vi "SwissSPAD Live_Pre-Recording Checks.vi"(8 "error in (no error)":errorcluster, 9 "Init Series?":bool, 11 "SwissSPAD Live Internal Variables in":T1={"okCFrontPanelDevices Refnum"=refnum, "Bottom Device Refnum"=refnum, "Display Image"=refnum, "# Live Images"=0, "relative s"=0.0, "# Image Sets"=0, "Message"="", "Current Image Set"=0, "# Datasets in Series"=0, "Current Dataset"=0, "Live Mode"=FALSE, "Recording Mode"=FALSE, "Record Button"=refnum, "\nLive Button"=refnum, "SwissSPAD Live Gate Image Data Q Name"="SS2 Live Gate Data Q", "Discard First Image"=FALSE, "Image Information"={"Save ROI Only"=FALSE, "Left"=0, "Top"=0, "Right"=0, "Bottom"=0, "Use Current ROI"=FALSE}, "Image Binning Options"={"Use Image Binning"=FALSE, "X Bin"=1, "Y Bin"=1}, "Bottom FPGA Serial Number"="", "Detector PCB Version"=enum."SS2 PCB1", "# Acquisitions"=1, "10 bits"=FALSE, "Top FPGA Serial Number"="", "Top Device Refnum"=refnum, "okCFrontPanel Refnum"=refnum} {"# Acquisitions" min=1; "Image Binning Options"."Y Bin" min=1; "Image Binning Options"."X Bin" min=1}) -> (0 "error out":errorcluster, 1 "Message":string, 2 "Ready?":bool, 3 "SwissSPAD Live Internal Variables out":T1={"okCFrontPanelDevices Refnum"=refnum, "Bottom Device Refnum"=refnum, "Display Image"=refnum, "# Live Images"=0, "relative s"=0.0, "# Image Sets"=0, "Message"="", "Current Image Set"=0, "# Datasets in Series"=0, "Current Dataset"=0, "Live Mode"=FALSE, "Recording Mode"=FALSE, "Record Button"=refnum, "\nLive Button"=refnum, "SwissSPAD Live Gate Image Data Q Name"="SS2 Live Gate Data Q", "Discard First Image"=FALSE, "Image Information"={"Save ROI Only"=FALSE, "Left"=0, "Top"=0, "Right"=0, "Bottom"=0, "Use Current ROI"=FALSE}, "Image Binning Options"={"Use Image Binning"=FALSE, "X Bin"=1, "Y Bin"=1}, "Bottom FPGA Serial Number"="", "Detector PCB Version"=enum."SS2 PCB1", "# Acquisitions"=1, "10 bits"=FALSE, "Top FPGA Serial Number"="", "Top Device Refnum"=refnum, "okCFrontPanel Refnum"=refnum} {"# Acquisitions" min=1; "Image Binning Options"."Y Bin" min=1; "Image Binning Options"."X Bin" min=1}, 4 "Verbose Message":string)   [LabVIEW 2021]
uses:
  SwissSPAD Live_Internal Variables.ctl
  D:/UCLA Thinkpad Google Drive/LabVIEW 2021 SP1/builds/SwissSPAD Live Distribution/Opal Kelly/C# Wrapper/v5.0.2/libFrontPanel-csharp.dll
  Opal Kelly/C# Wrapper/v5.0.2/libFrontPanel-csharp.dll
  <vilib>/vision/Image Controls.llb/IMAQ Image.ctl
  SwissSPAD Live_Image ROI Information.ctl
  Phasor/Image Binning Options.ctl
  SwissSPAD Live_SSx PCB Version.ctl
  SwissSPAD Live_Settings List.ctl
  SwissSPAD Live_File Information.ctl
  SwissSPAD Live_Globals.vi
  Variant/Variant to Data/Variant to Data.lvlib
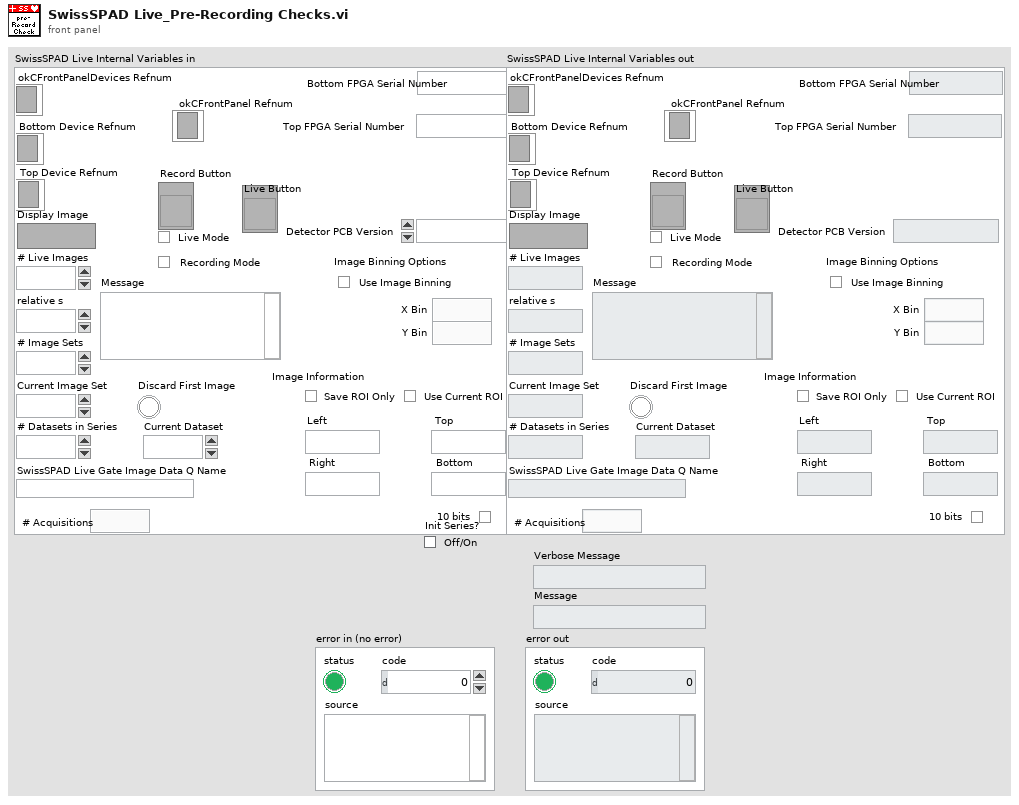
[diagram p1: front panel]
types:
  T1 = typedef "SwissSPAD Live_Internal Variables.ctl" = cluster{"okCFrontPanelDevices Refnum":refnum<k24>, "Bottom Device Refnum":refnum<k24>, "Display Image":T2, "# Live Images":i32, "relative s":dbl, "# Image Sets":i32, "Message":string, "Current Image Set":i32, "# Datasets in Series":i32, "Current Dataset":i32, "Live Mode":bool, "Recording Mode":bool, "Record Button":refnum<vi>, "\nLive Button":refnum<vi>, "SwissSPAD Live Gate Image Data Q Name":string, "Discard First Image":bool, "Image Information":T3, "Image Binning Options":T4, "Bottom FPGA Serial Number":string, "Detector PCB Version":T5, "# Acquisitions":u32, "10 bits":bool, "Top FPGA Serial Number":string, "Top Device Refnum":refnum<k24>, "okCFrontPanel Refnum":refnum<k24>}
  T2 = typedef "IMAQ Image.ctl" = refnum<image>
  T3 = typedef "SwissSPAD Live_Image ROI Information.ctl" = cluster{"Save ROI Only":bool, "Left":u16, "Top":u16, "Right":u16, "Bottom":u16, "Use Current ROI":bool}
  T4 = typedef "Image Binning Options.ctl" = cluster{"Use Image Binning":bool, "X Bin":i32, "Y Bin":i32}
  T5 = typedef "SwissSPAD Live_SSx PCB Version.ctl" = enum16{"unknown", "SS2 PCB1", "SS2 PCB2", "SS3 PCB1"}
  T6 = typedef "SwissSPAD Live_Settings List.ctl" = enum16{"FPGA:Bottom Half", "FPGA:Top Half", "FPGA:Bottom Bitfile Path", "FPGA:Top Bitfile Path", "FPGA:Bottom Bitstream Version", "FPGA:Top Bitstream Version", "FPGA:Auto Reset FPGA", "FPGA:Bottom FPGA Serial Number", "FPGA:Top FPGA Serial Number", "FPGA:Detector PCB Version", "Acquisition Parameters:Microlens", "Acquisition Parameters:SS2 DAQ Parameters", "Acquisition Parameters:Gate Configuration Array", "Acquisition Parameters:SS3 DAQ Parameters", "Acquisition Parameters:Buffer Size (# 8-bit Gates)", "File Information:File Information", "File Information:# Datasets in Series", "File Information:Scrambled File Flag", "File Information:SS3 Gate Slip Correction", "File Information:SS3 Hot Pixel Mismatch Detection", "File Information:Delay between Datasets", "File Information:Save Sum of All Gates Preview", "Image Parameters:Image ROI Information", "Image Parameters:Image Binning Options", "Image Parameters:SS3 Displayed Image", "Image Parameters:Image Display Options", "Image Parameters:Use Histogram Cursors", "Image Parameter:FPGA Data to Display", "UI Settings:Histogram Bins Number", "UI Settings:Histogram Bin Size", "UI Settings:Use Image Display Options", "UI Settings:Verbose Settings", "UI Settings:Verbose Saving"}
  T7 = typedef "SwissSPAD Live_File Information.ctl" = cluster{"File Folder":path, "File Name":string, "File Index":u32, "Author":string, "Sample":string, "Compression":bool, "Compression Level":u8}
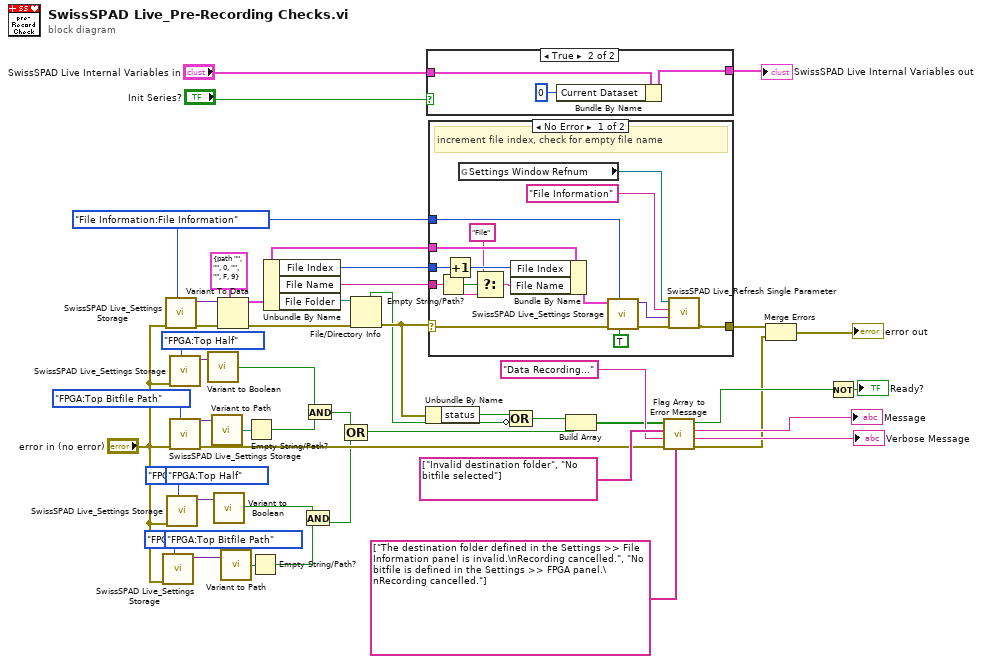
[diagram p0: block diagram]
diagram:
  (unwired) SwissSPAD_Live_Settings_List."FPGA:Top Half" ("Settings List")
  (unwired) SwissSPAD_Live_Settings_List."FPGA:Top Bitfile Path" ("Settings List")
  (unwired) SwissSPAD_Live_Settings_List."FPGA:Top Half" ("Settings List")
  w10 = SwissSPAD_Live_Settings_List."File Information:File Information" ("Settings List")
  n1 = call "SwissSPAD Live_Settings Storage.vi"("Settings List"=SwissSPAD_Live_Settings_List."FPGA:Bottom Bitfile Path", "Error In"="error in (no error)") -> ("Variant Data out"=w1:variant)  [unwired: 8 in, 1 out]
  n2 = call "SwissSPAD Live_Settings Storage.vi"("Settings List"=w10, "Error In"="error in (no error)") -> ("Error Out"=w45:errorcluster, "Variant Data out"=w3:variant)  [unwired: 8 in]
  n3 = call "SwissSPAD Live_Settings Storage.vi"("Settings List"=SwissSPAD_Live_Settings_List."FPGA:Bottom Half", "Error In"="error in (no error)") -> ("Variant Data out"=w2:variant)  [unwired: 8 in, 1 out]
  n4 = call "SwissSPAD Live_Settings Storage.vi"("Settings List"=SwissSPAD_Live_Settings_List."FPGA:Top Half", "Error In"="error in (no error)") -> ("Variant Data out"=w4:variant)  [unwired: 8 in, 1 out]
  n5 = call "SwissSPAD Live_Settings Storage.vi"("Settings List"=SwissSPAD_Live_Settings_List."FPGA:Top Bitfile Path", "Error In"="error in (no error)") -> ("Error Out"=w26:errorcluster, "Variant Data out"=w5:variant)  [unwired: 8 in]
  n6 = call "Variant to Boolean.vi"("Variant"=w4) -> ("Value"=w19:bool)  [unwired: 8 in]
  n7 = call "Variant to Path.vi"("Variant"=w5) -> ("Path"=w46:path)  [unwired: 8 in]
  n8 = call "Variant to Boolean.vi"("Variant"=w2) -> ("Value"=w11:bool)  [unwired: 8 in]
  n9 = Variant To Data(error in=w45, type=T7 {"File Folder"=path "", "File Name"="", "File Index"=0, "Author"="", "Sample"="", "Compression"=FALSE, "Compression Level"=9} ("File Information"), Variant=w3) -> (data=w40:T7, error out=w42:errorcluster)
  n10 = call "Variant to Path.vi"("Variant"=w1) -> ("Path"=w16:path)  [unwired: 8 in]
  n11 = Empty String/Path?(string/path=w46) -> (empty?=w18:bool)
  n12 = Empty String/Path?(string/path=w16) -> (empty?=w17:bool)
  n13 = Unbundle By Name(w40) -> ("File Index"=w41:u32, "File Name"=w39:string, "File Folder"=w43:path)
  n14 = And(x=w11, y=w17) -> (x .and. y?=w14:bool)
  n15 = And(x=w19, y=w18) -> (x .and. y?=w15:bool)
  n16 = Compound Arithmetic op=OR(w15, w14) -> (w13:bool)
  n17 = File/Directory Info(path=w43, error in=w42) -> (directory=w35:bool, error out=w38:errorcluster)  [unwired: 5 out]
  n18 = Unbundle By Name(w38) -> ("status"=w36:bool)
  n19 = case shown="True" "Init Series?" {
    tunnel: "SwissSPAD Live Internal Variables in" -> [w47 w50]
    tunnel: [w47 w49] -> w20
    frame False {
    }
    frame True {
      n20 = Bundle By Name(cluster=w50, "Current Dataset"=0) -> (w49:T1)
    }
  }
  "SwissSPAD Live Internal Variables out" <- w20
  n21 = case shown="No Error" w38 {
    selector: w38 -> [w63 w67]
    tunnel: w41 -> [w65 _]
    tunnel: w40 -> [w66 _]
    tunnel: w39 -> [w59 _]
    tunnel: w10 -> [w52 _]
    tunnel: [w56 w67] -> w23
    frame No Error {
      # "increment file index, check for empty file name"
      n22 = Empty String/Path?(string/path=w59) -> (empty?=w61:bool)
      n23 = Increment(x=w65) -> (x+1=w64:u32)
      n24 = global read "SwissSPAD Live_Globals.vi" "Settings Window Refnum"() -> (w55:refnum<vi>)
      n25 = Select(t="File", s=w61, f=w59) -> (s? t:f=w60:string)
      n26 = Bundle By Name(cluster=w66, "File Index"=w64, "File Name"=w60) -> (w53:T7)
      n27 = call "SwissSPAD Live_Settings Storage.vi"("Set/Get(F)"=TRUE, "Settings List"=w52, "Error In"=w63, "Variant Data in"=w53) -> ("Error Out"=w57:errorcluster, "Variant Data out"=w51:variant)  [unwired: 6 in]
      n28 = call "SwissSPAD Live_Refresh Single Parameter.vi"("Error In"=w57, "Data"=w51, "Control Label"="File Information", "VI Ref in"=w55) -> ("Error Out"=w56:errorcluster)  [unwired: 7 in]
    }
    frame Error {
    }
  }
  n29 = Compound Arithmetic op=OR(w36, invert w35) -> (w32:bool)
  n30 = Build Array(w32, w13) -> (w31:bool[])
  n31 = call "Flag Array to Error Message.vi"("Verbose Message Array"=string[] ["The destination folder defined in the Settings >> File Information panel is invalid.\nRecording cancelled.", "No bitfile is defined in the Settings >> FPGA panel.\nRecording cancelled."], "Error In"=w26, "OK Message"="Data Recording..." ("f"), "Message Array"=string[] ["Invalid destination folder", "No bitfile selected"], "Flag Array"=w31) -> ("Error Out"=w25:errorcluster, "Verbose Message"=→"Verbose Message":string, "Message"=→"Message":string, "Flag OR"=w27:bool)  [unwired: 3 in]
  n32 = Merge Errors(w23, w25) -> (→"error out":errorcluster)
  n33 = Not(x=w27) -> (.not. x?=→"Ready?":bool)
